vi "InitDM_STED.vi"(11 "BM Flat":bool) -> (2 "IDs":i32[](array[numeric]), 3 "reference out":refnum<k7>)   [LabVIEW 2014]
uses:
  <vilib>/Utility/file.llb/Read From Spreadsheet File (DBL).vi
  <vilib>/Utility/file.llb/Read From Spreadsheet File (string).vi
  <vilib>/Analysis/Matrix/Numeric/Conversions/Array To Matrix - RA2.vi
  <vilib>/Analysis/Matrix/NI_Matrix.lvlib
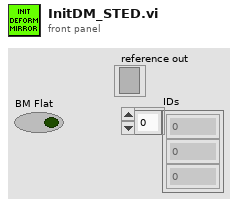
[diagram p1: front panel]
types:
  T1 = typedef "NI_Matrix.lvlib/RealMatrix.ctl" = dbl[][]
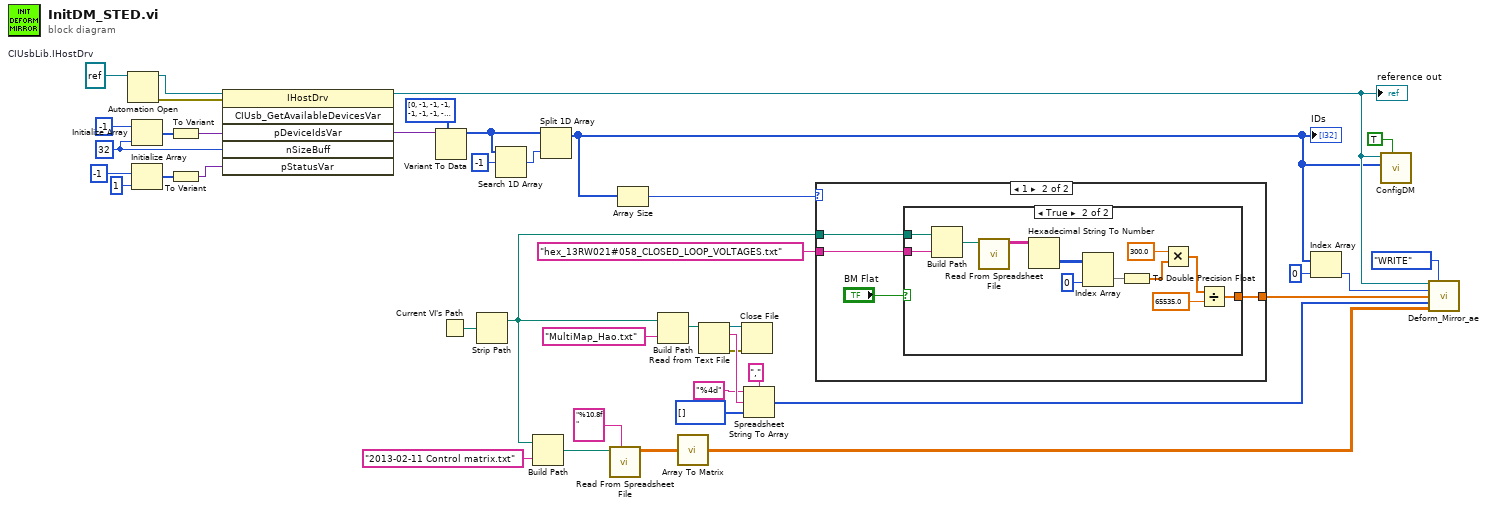
[diagram p0: block diagram]
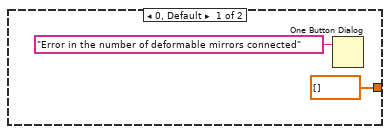
[diagram p2: hidden frame]
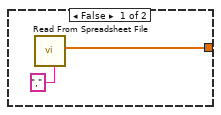
[diagram p3: hidden frame]
diagram:
  w36 = 32 ("dimension size")
  w27 = refnum<k7> refnum  # CIUsbLib.IHostDrv
  n1 = Automation Open(Automation Refnum=w27) -> (Automation Refnum=w32:refnum<k7>, error out=w33:errorcluster)  [unwired: 1 in, 2 out]
  n2 = Initialize Array(-1 ("element"), w36) -> (w29:i32[])
  n3 = Initialize Array(-1 ("element"), 1 ("dimension size")) -> (w28:i32[])
  n4 = To Variant(anything=w29) -> (Variant=w30:variant)
  n5 = To Variant(anything=w28) -> (Variant=w35:variant)
  n6 = invoke class="IHostDrv" method="CIUsb_GetAvailableDevicesVar"(reference=w32, error in=w33, "pDeviceIdsVar"=w30, "nSizeBuff"=w36, "pStatusVar"=w35) -> (reference out=w7:refnum<k7>, "pDeviceIdsVar"=w41:variant)  [unwired: 1 in, 4 out]
  "reference out" <- w7
  n7 = Variant To Data(type=i32[] [0, -1, -1, -1, -1, -1, -1, -1, -1, -1, -1, -1, -1, -1, -1, -1, -1, -1, -1, -1, -1, -1, -1, -1, -1, -1, -1, -1, -1, -1, -1, -1] ("pDeviceIDs"), Variant=w41) -> (data=w39:i32[])  [unwired: 1 in, 1 out]
  n8 = Current VI's Path() -> (path=w22:path)
  n9 = Strip Path(path=w22) -> (stripped path=w14:path)  [unwired: 1 out]
  n10 = Search 1D Array(1D array=w39, element=-1) -> (index of element=w38:i32)  [unwired: 1 in]
  n11 = Build Path(base path=w14, name or relative path="2013-02-11 Control matrix.txt") -> (appended path=w15:path)
  n12 = Split 1D Array(array=w39, index=w38) -> (first subarray=w6:i32[])  [unwired: 1 out]
  "IDs" <- w6
  n13 = call-poly <vilib>:"Read From Spreadsheet File.vi"("format (%.3f)"="%10.8f", "file path (dialog if empty)"=w15) -> ("all rows"=w4:dbl[][])  [unwired: 2 in, 7 out]
  n14 = Array Size(array=w6) -> (size(s)=w12:i32)
  n15 = Build Path(base path=w14, name or relative path="MultiMap_Hao.txt") -> (appended path=w19:path)
  n16 = call-poly <vilib>:"Array To Matrix.vi"("Real 2D Array"=w4) -> ("Real Matrix"=w11:T1)
  n17 = Read from Text File(file (use dialog)=w19) -> (refnum out=w21:refnum<file>, text=w26:string, error out=w20:errorcluster)  [unwired: 1 in, 3 out]
  n18 = Close File(refnum=w21, error in=w20) -> ()  [unwired: 2 out]
  n19 = Spreadsheet String To Array(delimiter (Tab)=",", format string="%4d", spreadsheet string=w26, array type (2D Dbl)=i32[] []) -> (array=w9:i32[])
  n20 = case shown="1" w12 {
    tunnel: w14 -> [_ w47]
    tunnel: "hex_13RW021#058_CLOSED_LOOP_VOLTAGES.txt" ("name or relative path") -> [_ w46]
    tunnel: [dbl[] [] w45] -> w1
    frame 0, Default {
      n21 = One Button Dialog(message="Error in the number of deformable mirrors connected") -> ()  [unwired: 1 in, 1 out]
    }
    frame 1 {
      n22 = case shown="True" "BM Flat" {
        tunnel: w47 -> [_ w61]
        tunnel: w46 -> [_ w60]
        tunnel: [w48 w51] -> w45
        frame False {
          n23 = call-poly <vilib>:"Read From Spreadsheet File.vi"("delimiter (\\t)"="," ("delimiter (\\t)")) -> ("first row"=w48:dbl[])  [unwired: 6 in, 4 out]
        }
        frame True {
          n24 = Build Path(base path=w61, name or relative path=w60) -> (appended path=w59:path)
          n25 = call-poly <vilib>:"Read From Spreadsheet File.vi"("file path (dialog if empty)"=w59) -> ("all rows"=w58:string[][])  [unwired: 3 in, 7 out]
          n26 = Hexadecimal String To Number(string=w58) -> (number=w57:u32[][])  [unwired: 2 in, 1 out]
          n27 = Index Array(array=w57, index (col)=0 ("disabled index (col)")) -> (element=w55:u32[])  [unwired: 1 in]
          n28 = To Double Precision Float(number=w55) -> (double precision float=w50:dbl[])
          n29 = Multiply(x=300.0 ("y"), y=w50) -> (x*y=w54:dbl[])
          n30 = Divide(x=w54, y=65535.0) -> (x/y=w51:dbl[])
        }
      }
    }
  }
  n31 = Index Array(array=w6, index=0) -> (element=w3:i32)
  n32 = call "ConfigDM.vi"("High Voltage"=TRUE, "Dev IDs"=w6, "Automation Refnum in"=w7) -> ()  [unwired: 7 in, 2 out]
  n33 = call "Deform_Mirror_ae.vi"("Refnum In"=w7, "Enum"=enum16{"WRITE", "READ"}."WRITE", "IDs In"=w3, "Flat Files In"=w1, "Multi Map Data In"=w9, "Mode Matrix In"=w11) -> ()  [unwired: 5 in, 5 out]
